vi "Edge Detection with 2D Convolution.vi"() -> ()   [LabVIEW 2023]
doc: "This VI uses two-dimensional convolution to perform image edge detection."
uses:
  <vilib>/Analysis/Matrix/Datatypes/RealMatrix.ctl
  <vilib>/Analysis/2dsp.llb/2D Convolution (DBL).vi
  <vilib>/Analysis/NI_AALPro.lvlib
  <vilib>/Analysis/Matrix/NI_Matrix.lvlib
panel:
  out "Sum":dbl
  in  "Operator Type":u16(ring) items=["Laplacian Type I", "Laplacian Type II", "Arbitrary"]
  in  "Stop":bool
  out "Edge Image":dbl[][](graph)
  in  "Convolution Mask":T1=[[1.0, 1.0, 1.0], [1.0, -8.0, 1.0], [1.0, 1.0, 1.0]]
  in  "Image Selector":u16(ring) items=["Cameraman", "Couple", "Columbia", "Baboon"]
  out "Source Image":u8[][](graph)
  # "Overview: This VI uses two-dimensional convolution to perform image edge detection.\nRequirements: LabVIEW Full Development System\nInstructions: \n1. Run the VI and select an image with the Image Selector.\n2. Change the Operator Type and verify its effect on the Edge Image. Change Operator Type to \"Arbitrary\" and change the kernels by modifying the Convolution Mask. Notice that the sum of all the elements of the Convolution Mask should to be zero to apply the edge detection correctly.\n3. Click Stop to stop the VI."
  # "Convolution"
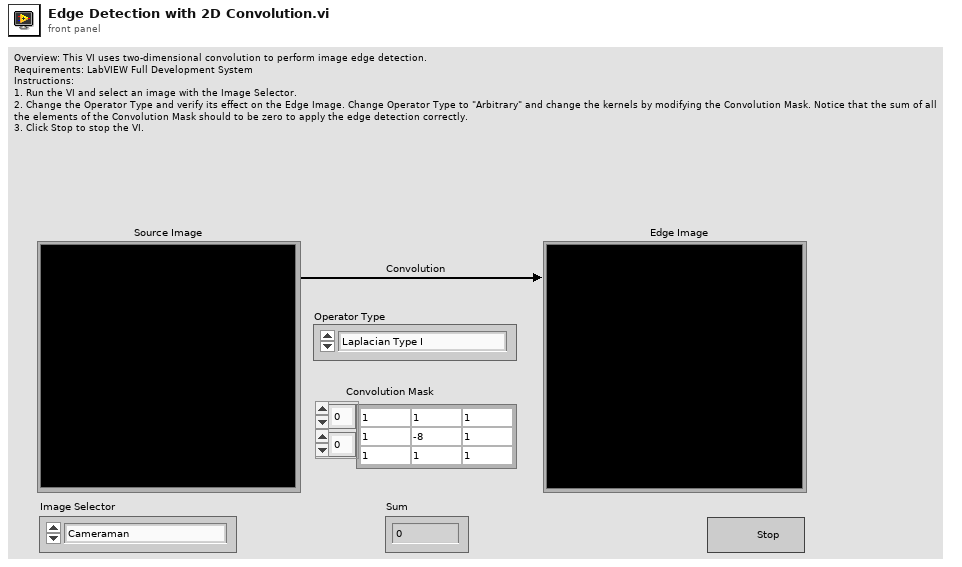
[diagram p1: front panel]
types:
  T1 = typedef "NI_Matrix.lvlib/RealMatrix.ctl" = dbl[][]
  T2 = enum8{"Enabled", "Disabled", "Disabled and Grayed Out"}
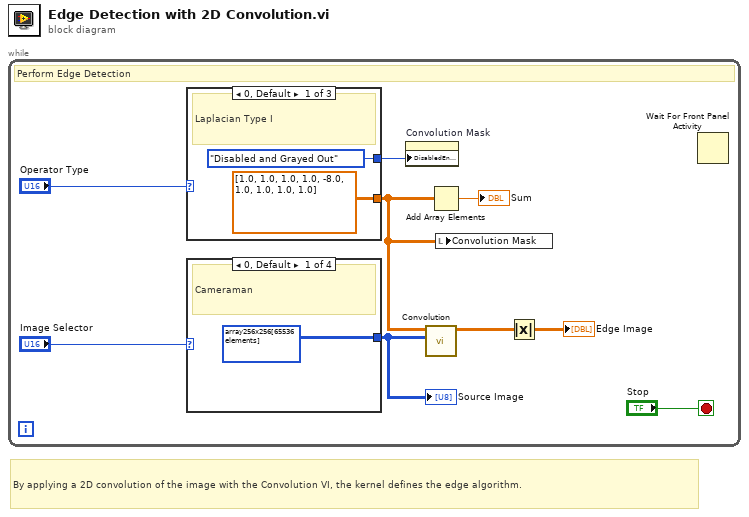
[diagram p0: block diagram]
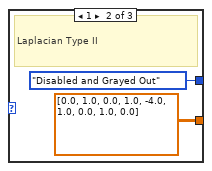
[diagram p2: hidden frame]
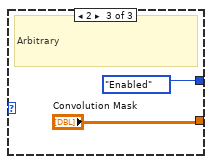
[diagram p3: hidden frame]
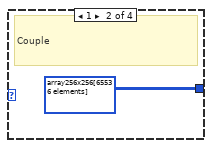
[diagram p4: hidden frame]
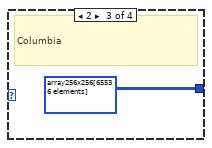
[diagram p5: hidden frame]
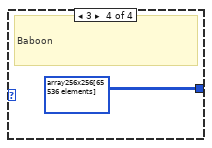
[diagram p6: hidden frame]
diagram:
  # "By applying a 2D convolution of the image with the Convolution VI, the kernel defines the edge algorithm."
  n1 = while {
    stop <- "Stop" stop-if-true
    # "Perform Edge Detection"
    n2 = case shown="0, Default" "Operator Type" {
      tunnel: [dbl[][] [[1.0, 1.0, 1.0], [1.0, -8.0, 1.0], [1.0, 1.0, 1.0]] dbl[][] [[0.0, 1.0, 0.0], [1.0, -4.0, 1.0], [0.0, 1.0, 0.0]] "Convolution Mask"] -> w2
      tunnel: [T2."Disabled and Grayed Out" ("Disabled") T2."Disabled and Grayed Out" ("Disabled") T2."Enabled" ("Disabled")] -> w1
      frame 0, Default {
        # "Laplacian Type I"
      }
      frame 1 {
        # "Laplacian Type II"
      }
      frame 2 {
        # "Arbitrary"
      }
    }
    n3 = case shown="0, Default" "Image Selector" {
      tunnel: [u8[][] array256x256[65536 elements] ("Image Pixels (U8)") u8[][] array256x256[65536 elements] ("Image Pixels (U8)") u8[][] array256x256[65536 elements] ("Image Pixels (U8)") u8[][] array256x256[65536 elements] ("Image Pixels (U8)")] -> w8
      frame 0, Default {
        # "Cameraman"
      }
      frame 1 {
        # "Couple"
      }
      frame 2 {
        # "Columbia"
      }
      frame 3 {
        # "Baboon"
      }
    }
    "Source Image" <- w8
    n4 = property on="Convolution Mask" class="Arr (strict)"("DisabledEnum"=w1) -> ()  [unwired: 2 in, 2 out]
    n5 = call-poly <vilib>:"Convolution.vi"("Y"=w8, "X"=w2) -> ("X * Y"=w7:dbl[][])  [unwired: 8 in, 1 out]
    n6 = Add Array Elements(numeric array=w2) -> (sum=→"Sum":dbl)
    n7 = local write "Convolution Mask"(w2) -> ()
    n8 = Absolute Value(x=w7) -> (abs(x)=→"Edge Image":dbl[][])
    n9 = Wait For Front Panel Activity() -> ()  [unwired: 3 in, 1 out]
  }
